vi "update_sleep_detection_parameters.vi"(4 "Input \nparameters":T2={"Frame rate (ms)"=2000, "Worm strain"="N2", "Time t"=0, "State"=enum."Image acquisition", "Time elapsed"=0.0, "Max_num_runs"=100000, "#TTL"=0, "Time of start TTL"=100000, "ImSub Value"=0, "Time of last TTL"=0, "Number of Columns"=2, "Number of Rows"=2, "# AdjacentTTL"=0, "Sleep deprivation status"="", "Sleep Detection"=FALSE, "# Sleep detections"=0, "Time of first sleep detection"=0, "Time max # adjacent TTL"=0, "Image t-1"=[], "Image t"=[]} {"Number of Rows" items=["1"=1, "2"=2, "3"=3, "4"=4]; "Number of Columns" items=["1"=1, "2"=2, "3"=3, "4"=4]}) -> (1 "Output \nParameters":T2={"Frame rate (ms)"=2000, "Worm strain"="N2", "Time t"=0, "State"=enum."Image acquisition", "Time elapsed"=0.0, "Max_num_runs"=100000, "#TTL"=0, "Time of start TTL"=100000, "ImSub Value"=0, "Time of last TTL"=0, "Number of Columns"=2, "Number of Rows"=2, "# AdjacentTTL"=0, "Sleep deprivation status"="", "Sleep Detection"=FALSE, "# Sleep detections"=0, "Time of first sleep detection"=0, "Time max # adjacent TTL"=0, "Image t-1"=[], "Image t"=[]} {"Number of Rows" items=["1"=1, "2"=2, "3"=3, "4"=4]; "Number of Columns" items=["1"=1, "2"=2, "3"=3, "4"=4]})   [LabVIEW 2011]
uses:
  state.ctl
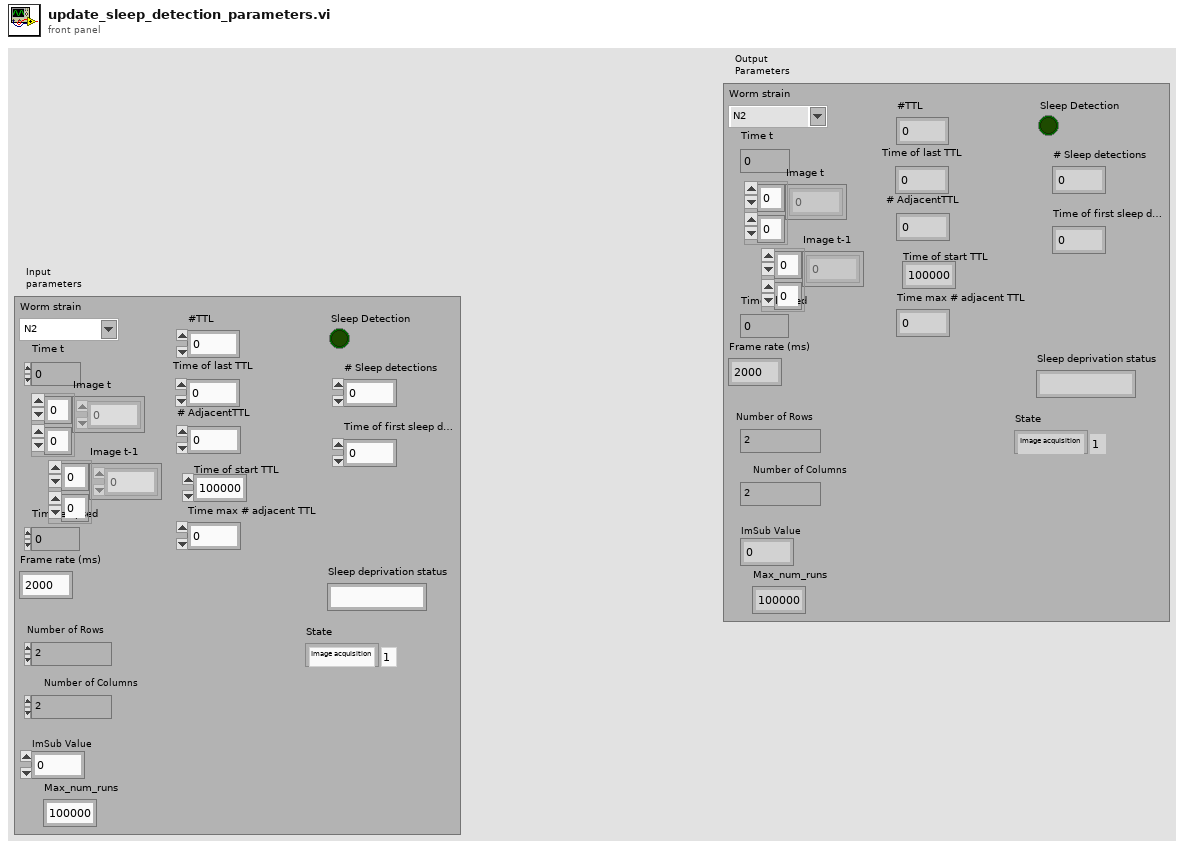
[diagram p1: front panel]
types:
  T1 = typedef "state.ctl" = enum16{"Initialize measurement", "Image acquisition", "Image processing", "Sleep detection", "Control TTL protocol ", "Sleep deprivation", "Update image & exit condition", "Wait "}
  T2 = cluster{"Frame rate (ms)":u32, "Worm strain":string, "Time t":i32, "State":T1, "Time elapsed":dbl, "Max_num_runs":i32, "#TTL":i32, "Time of start TTL":i32, "ImSub Value":i32, "Time of last TTL":i32, "Number of Columns":u32, "Number of Rows":u32, "# AdjacentTTL":i32, "Sleep deprivation status":string, "Sleep Detection":bool, "# Sleep detections":i32, "Time of first sleep detection":i32, "Time max # adjacent TTL":i32, "Image t-1":i32[][], "Image t":i32[][]}
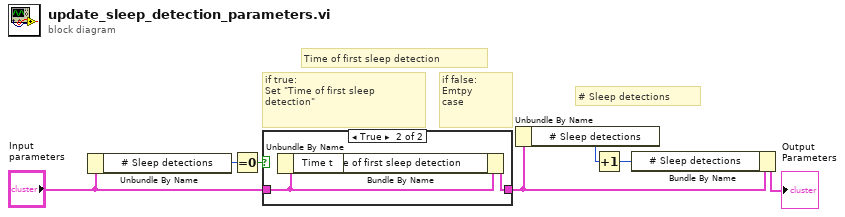
[diagram p0: block diagram]
diagram:
  # "Time of first sleep detection"
  # "if false:\nEmtpy \ncase"
  # "if true:\nSet \"Time of first sleep\ndetection\""
  # "# Sleep detections"
  n1 = Unbundle By Name("Input \nparameters") -> ("# Sleep detections"=w5:i32)
  n2 = Equal To 0?(x=w5) -> (x = 0?=w3:bool)
  n3 = case shown="True" w3 {
    tunnel: "Input \nparameters" -> [w8 w10]
    tunnel: [w8 w9] -> w2
    frame False {
    }
    frame True {
      n4 = Unbundle By Name(w10) -> ("Time t"=w11:i32)
      n5 = Bundle By Name(cluster=w10, "Time of first sleep detection"=w11) -> (w9:T2)
    }
  }
  n6 = Unbundle By Name(w2) -> ("# Sleep detections"=w7:i32)
  n7 = Increment(x=w7) -> (x+1=w6:i32)
  n8 = Bundle By Name(cluster=w2, "# Sleep detections"=w6) -> (→"Output \nParameters":T2)
